vi "Transfer Displacement Offsets.vi"(2 "error in":errorcluster) -> (0 "error out":errorcluster)   [LabVIEW 2013]
uses:
  Data Access Objects/Metadata/LBCB Number.ctl
  Global Data/Transactions/Dataset Type.ctl
  Global Data/Transactions/Dataset Transaction Id.ctl
  Global Data/Transactions/Dataset Source.ctl
  Apps/Yes No Button.ctl
  Data Access Objects/Metadata/Persistant DAO Actions.ctl
  LbcbConversions/LBCB_Conversions_Actions.ctl
  Data Access Objects/Metadata/DAO Actions with Remove.ctl
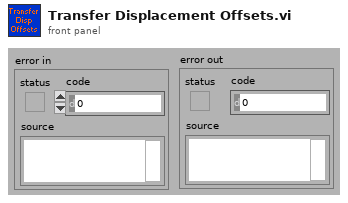
[diagram p1: front panel]
types:
  T1 = typedef "Dataset Transaction Id.ctl" = cluster{"Dataset Source":T2, "Dataset Type":T3, "Hold":T4, "Volts":T4, "Tag":string}
  T2 = typedef "Dataset Source.ctl" = enum16{"LBCB 1", "LBCB 2", "Combined", "External Sensors"}
  T3 = typedef "Dataset Type.ctl" = enum16{"LVDT", "Load Cell", "Actuator Command", "Servo Error", "Displacement Command", "Displacement", "Force"}
  T4 = typedef "Yes No Button.ctl" = bool
  T5 = typedef "LBCB Number.ctl" = enum16{"LBCB1", "LBCB2"}
  T6 = typedef "DAO Actions with Remove.ctl" = enum16{"Init", "Get", "Set", "Remove"}
  T7 = typedef "LBCB_Conversions_Actions.ctl" = enum16{"A2C", "C2A", "Set Log Filename", "Init"}
  T8 = typedef "Persistant DAO Actions.ctl" = enum16{"Init", "Get", "Set", "Load", "Save"}
  T9 = typedef "LBCB Position.ctl" = cluster{"Motion Center":dbl[], "Transformation Matrix":dbl[][]}
  T10 = typedef "LBCB Settings.ctl" = cluster{"Size":T11, "Type":T12}
  T11 = typedef "LBCB Size.ctl" = enum16{"1/5th-scale LBCB", "Full-scale LBCB", "Portable LBCB", "Mid-Scale LBCB"}
  T12 = typedef "LBCB Type.ctl" = enum16{"X Actuators On The Left", "X Actuators On The Right"}
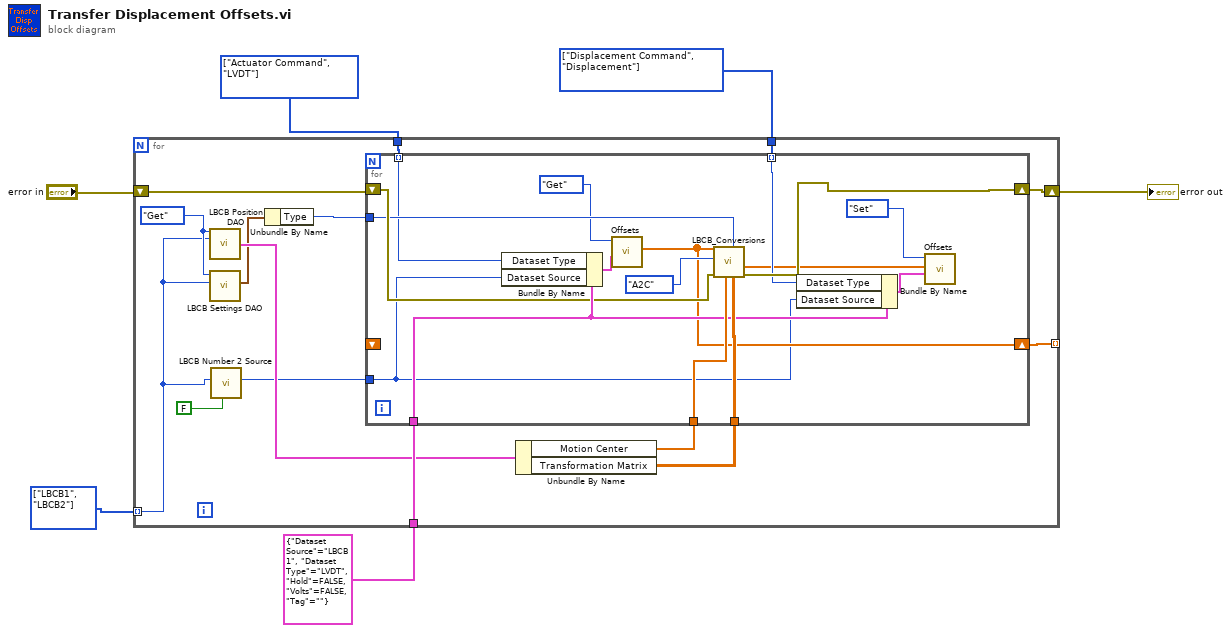
[diagram p0: block diagram]
diagram:
  w5 = T3[] [enum."Displacement Command", enum."Displacement"] items=["LVDT", "Load Cell", "Actuator Command", "Servo Error", "Displacement Command", "Displacement", "Force"]
  w6 = T3[] [enum."Actuator Command", enum."LVDT"] items=["LVDT", "Load Cell", "Actuator Command", "Servo Error", "Displacement Command", "Displacement", "Force"]
  w2 = T5[] [enum."LBCB1", enum."LBCB2"] items=["LBCB1", "LBCB2"]
  n1 = for {
    shift-right: [w17] -> w4
    shift-left: "error in" -> [w19]
    tunnel: w6 -> [w16]
    tunnel: w5 -> [w15]
    tunnel: w2 -> [w9] mode=indexing
    tunnel: T1 {"Dataset Source"=enum."LBCB 1", "Dataset Type"=enum."LVDT", "Hold"=FALSE, "Volts"=FALSE, "Tag"=""} ("Dataset Trans Id") -> [w14]
    tunnel: [w10] -> _ mode=indexing
    w13 = Persistant_DAO_Actions."Get" ("LBCB Settings Actions")
    n2 = call "LBCB Position DAO.vi"("LBCB Settings Actions"=w13, "LBCB Number"=w9) -> ("LBCB Position Output"=w12:T9)  [unwired: 11 in, 2 out]
    n3 = call "LBCB Settings DAO.vi"("LBCB Number"=w9, "Actions"=w13) -> ("LBCB Setting Out"=w11:T10)  [unwired: 7 in, 2 out]
    n4 = call "LBCB Number 2 Source.vi"("Combined"=FALSE, "LBCB Number"=w9) -> ("Dataset Source"=w8:T2)  [unwired: 9 in]
    n5 = Unbundle By Name(w11) -> ("Type"=w18:T12)
    n6 = Unbundle By Name(w12) -> ("Motion Center"=w21:dbl[], "Transformation Matrix"=w20:dbl[][])
    n7 = for {
      tunnel: w21 -> [w37]
      tunnel: w20 -> [w36]
      tunnel: w14 -> [w35]
      tunnel: w18 -> [w33]
      tunnel: w16 -> [w30] mode=indexing
      shift-right: [w32] -> w17
      shift-left: w19 -> [w34]
      tunnel: w15 -> [w31] mode=indexing
      shift-right: [w23] -> w10
      shift-left: _ -> [_]
      tunnel: w8 -> [w22]
      n8 = Bundle By Name(cluster=w35, "Dataset Type"=w30, "Dataset Source"=w22) -> (w28:T1)
      n9 = call "Offsets.vi"("Dataset Trans Id"=w28, "DAO Actions"=DAO_Actions_with_Remove."Get") -> ("Data Out"=w23:dbl[])  [unwired: 7 in, 2 out]
      n10 = call "LBCB_Conversions.vi"("Transformation Matrix"=w36, "Type"=w33, "Motion Center"=w37, "error in (no error)"=w34, "Conversion Type"=LBCB_Conversions_Actions."A2C", "Input"=w23) -> ("error out"=w32:errorcluster, "Output"=w24:dbl[])  [unwired: 4 in]
      n11 = Bundle By Name(cluster=w35, "Dataset Type"=w31, "Dataset Source"=w22) -> (w27:T1)
      n12 = call "Offsets.vi"("Dataset Trans Id"=w27, "Data In"=w24, "DAO Actions"=DAO_Actions_with_Remove."Set") -> ()  [unwired: 6 in, 3 out]
    }
  }
  "error out" <- w4
